vi "PH_SRDG645.get Trigger.vi"(0 "i ref in":refnum<vi>, 5 "error IO":errorcluster) -> (14 "i ref out":refnum<vi>, 19 "error out":errorcluster)   [LabVIEW 2014, in "PH_SRDG645.lvlib"]
doc: "This VI querries the trigger settings from the hardware."
uses:
  PH_SRDG645.lvlib
  PH_SRDG645.Trigger.ctl
  instr.lib/SRDG645/Stanford Research DG645 - Driver.lvlib
panel:
  in  "Trigger cluster":T1={"Source"=0, "Rate [Hz]"=1000.0, "Level [V]"=1.0} {"Rate [Hz]" format="%#_9p"; "Source" items=["Internal", "External rising edge", "External falling edge", "Single shot external rising edges", "Single shot external falling edges", "Single shot", "Line"]}
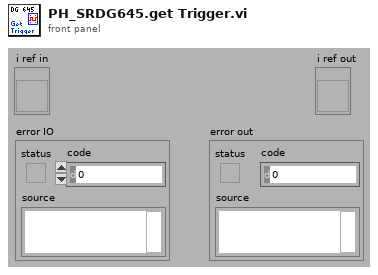
[diagram p1: front panel]
types:
  T1 = typedef "PH_SRDG645.lvlib/PH_SRDG645.Trigger.ctl" = cluster{"Source":i32, "Rate [Hz]":dbl, "Level [V]":dbl}
  T2 = typedef "PH_SRDG645.lvlib/PH_SRDG645.i attribute.ctl" = cluster{"GUI Refs":cluster{"Delete":refnum<vi>, "Device Errors":refnum<vi>, "Trigger":refnum<vi>, "Default Name":refnum<vi>, "Firmware Revision":refnum<vi>, "Serial Number":refnum<vi>, "Model":refnum<vi>, "Visa resource name":refnum<vi>}, "Service ID Rate":i32, "Service IDs Channelinfo":i32[], "VISA resource name":refnum<visa-resource-name>, "Device Errors":cluster{"code":i32, "Text":string}[], "Trigger":T1, "Channels":cluster{"T1":T3, "A":T3, "B":T3, "C":T3, "D":T3, "E":T3, "F":T3, "G":T3, "H":T3}, "GUI Refs Channels":refnum<vi>[], "Outputs":cluster{"AB":cluster{"Level Offset [V]":dbl, "Amplitue [V]":dbl, "Polarity":i32}, "CD":cluster{"Level Offset [V]":dbl, "Amplitue [V]":dbl, "Polarity":i32}, "EF":cluster{"Level Offset [V]":dbl, "Amplitue [V]":dbl, "Polarity":i32}, "GH":cluster{"Level Offset [V]":dbl, "Amplitue [V]":dbl, "Polarity":i32}, "T0":cluster{"Level Offset [V]":dbl, "Amplitue [V]":dbl, "Polarity":i32}}, "GUI Refs Outputs":refnum<vi>[], "Serial Number":string, "Firmweare Revision":string, "Model":string}
  T3 = typedef "PH_SRDG645.lvlib/PH_SRDG645.Channel Settings.ctl" = cluster{"Delay [s]":dbl, "relative to":i32}
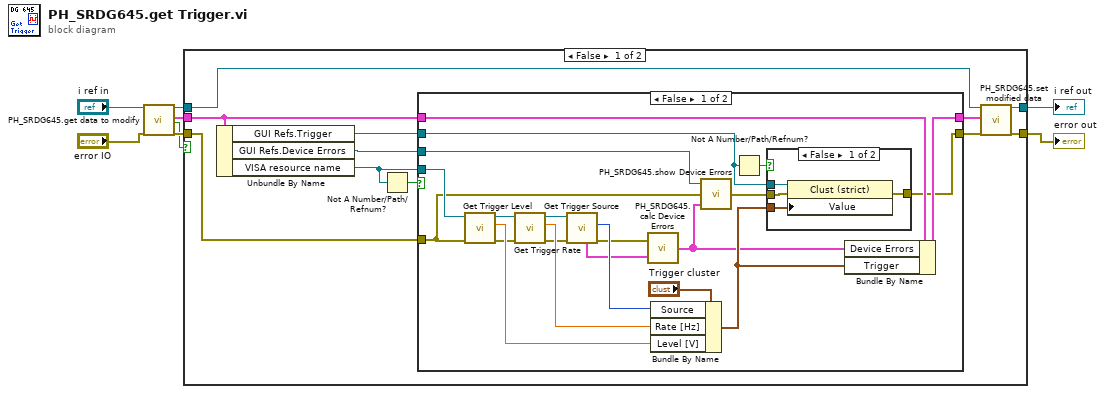
[diagram p0: block diagram]
diagram:
  n1 = call "PH_SRDG645.get data to modify.vi"("i ref in"="i ref in", "error in (no error)"="error IO") -> ("i ref out"=w6:refnum<vi>, "i attribute"=w3:T2, "timed out"=w1:bool, "error out"=w4:errorcluster)  [unwired: 14 in]
  n2 = case shown="False" w1 {
    tunnel: w6 -> [w11 w49]
    tunnel: [w19 w49] -> w5
    tunnel: w4 -> [w18 w48]
    tunnel: w3 -> [w17 _]
    tunnel: [w15 w48] -> w2
    frame False {
      n3 = Unbundle By Name(w17) -> ("GUI Refs.Trigger"=w13:refnum<vi>, "GUI Refs.Device Errors"=w12:refnum<vi>, "VISA resource name"=w9:refnum<visa-resource-name>)
      n4 = Not A Number/Path/Refnum?(number/path/refnum=w9) -> (NaN/Path/Refnum?=w10:bool)
      n5 = case shown="False" w10 {
        tunnel: w9 -> [w34 _]
        tunnel: w18 -> [w20 w46]
        tunnel: w17 -> [w31 w47]
        tunnel: [w30 w47] -> w16
        tunnel: [w28 w46] -> w14
        tunnel: w13 -> [w26 _]
        tunnel: w12 -> [w25 _]
        frame False {
          n6 = call "Get Trigger Level.vi"("error in (no error)"=w20, "VISA resource name"=w34) -> ("error out"=w36:errorcluster, "Trigger Level [V]"=w37:dbl, "VISA resource name out"=w33:refnum<visa-resource-name>)  [unwired: 6 in, 1 out]
          n7 = call "Get Trigger Rate.vi"("error in (no error)"=w36, "VISA resource name"=w33) -> ("error out"=w35:errorcluster, "Trigger Rate [Hz]"=w38:dbl, "VISA resource name out"=w32:refnum<visa-resource-name>)  [unwired: 6 in, 1 out]
          n8 = call "Get Trigger Source.vi"("error in (no error)"=w35, "VISA resource name"=w32) -> ("error out"=w24:errorcluster, "Trigger Source"=w39:i32, "Device Errors"=w23:cluster{"code":i32, "Text":string}[])  [unwired: 6 in, 1 out]
          n9 = call "PH_SRDG645.calc Device Errors.vi"("Device Errors out"=w23, "SRDG 645 error out"=w24) -> ("calculate Device Errors"=w22:cluster{"code":i32, "Text":string}[])
          n10 = Bundle By Name(cluster="Trigger cluster", "Source"=w39, "Rate [Hz]"=w38, "Level [V]"=w37) -> (w29:T1)
          n11 = call "PH_SRDG645.show Device Errors.vi"("Device Errors"=w22, "error in"=w20, "Ref Device Errors"=w25) -> ("error out"=w21:errorcluster)
          n12 = Not A Number/Path/Refnum?(number/path/refnum=w26) -> (NaN/Path/Refnum?=w27:bool)
          n13 = case shown="False" w27 {
            tunnel: w26 -> [w44 _]
            tunnel: w29 -> [w43 _]
            tunnel: [w42 w45] -> w28
            tunnel: w21 -> [w41 w45]
            frame False {
              n14 = property class="Clust (strict)"(reference=w44, error in=w41, "Value"=w43) -> (error out=w42:errorcluster)  [unwired: 1 out]
            }
            frame True {
            }
          }
          n15 = Bundle By Name(cluster=w31, "Device Errors"=w22, "Trigger"=w29) -> (w30:T2)
        }
        frame True {
        }
      }
      n16 = call "PH_SRDG645.set modified data.vi"("i ref in"=w11, "i attribute"=w16, "error in (no error)"=w14) -> ("i ref out"=w19:refnum<vi>, "error out"=w15:errorcluster)  [unwired: 15 in]
    }
    frame True {
    }
  }
  "error out" <- w2
  "i ref out" <- w5
